vi "UTIL_5PtCalibrate.vi"(11 "Digital in":refnum<vi>) -> (3 "Input":string)   [LabVIEW 2024]
panel:
  in  "Cal SP":dbl[](array[numeric])
  in  "Array":dbl[][](array[numeric])
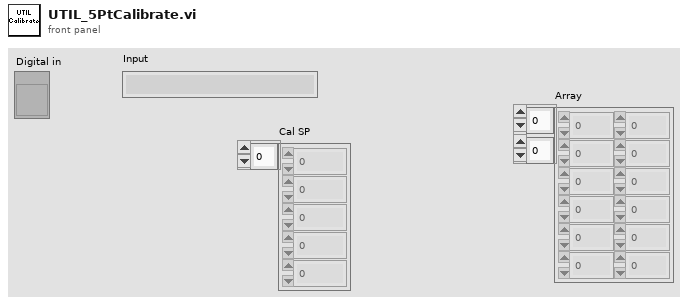
[diagram p1: front panel]
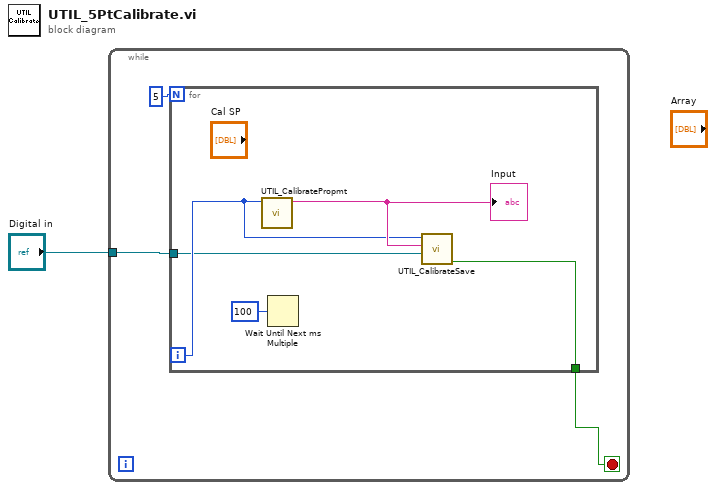
[diagram p0: block diagram]
diagram:
  n1 = while {
    tunnel: "Digital in" -> [w4]
    stop <- w2 stop-if-true
    n2 = for {
      N: 5 -> [_]
      tunnel: w4 -> [w6]
      tunnel: [w5] -> w2
      i -> [w7]
      n3 = call "UTIL_CalibratePropmt.vi"("Sequence"=w7) -> ("Input Out"=w8:string)  [unwired: 10 in]
      "Input" <- w8
      n4 = Wait Until Next ms Multiple(millisecond multiple=u32 100) -> ()  [unwired: 1 out]
      n5 = call "UTIL_CalibrateSave.vi"("Level Raw Refnum"=w6, "Input"=w8, "Sequence"=w7) -> ("T button?"=w5:bool)  [unwired: 8 in]
    }
  }
